vi "CheckExit.vi"(8 "error in":errorcluster, 11 "Car Position Slider":u16(slide) scale=0.0..10.0) -> (0 "error out":errorcluster, 3 "check":bool)   [LabVIEW 2020]
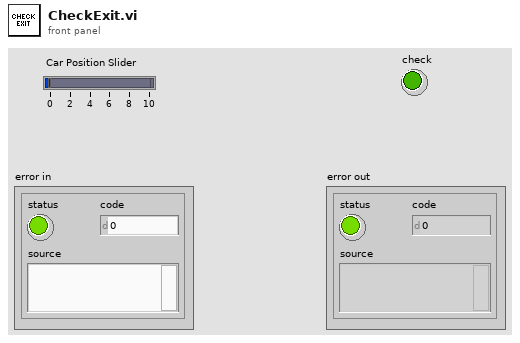
[diagram p1: front panel]
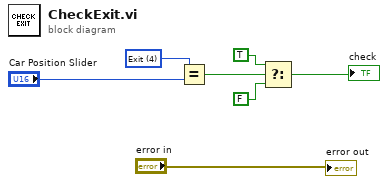
[diagram p0: block diagram]
diagram:
  w7 = u16 4 items=["Entry", "Station 1", "Station 2", "Station 3", "Exit"] ("Car Position Slider")
  n1 = Equal?(x=w7, y="Car Position Slider") -> (x = y?=w5:bool)
  n2 = Select(t=TRUE ("Wash Entry 2"), s=w5, f=FALSE ("Wash Entry 2")) -> (s? t:f=→"check":bool)
  "error out" <- "error in"
